vi "ctx get rssi value.vi"(9 "dest":u32, 10 "device_id":u32, 11 "context":u32) -> (1 "dest out":u32, 2 "function return":i32, 3 "context out":u32)   [LabVIEW 2019, in "apdm.lvlib"]
doc: "APDM_EXPORT int apdm_ctx_get_rssi_value(apdm_ctx_t context, const uint32_t device_id, uint32_t *dest);"
uses:
  apdm.lvlib
  Lee Lab/CP FES Walking 2018/Code/Working/LabVIEW/apdm.dll
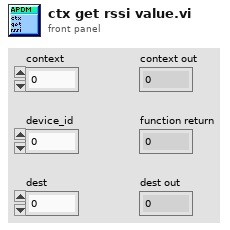
[diagram p1: front panel]
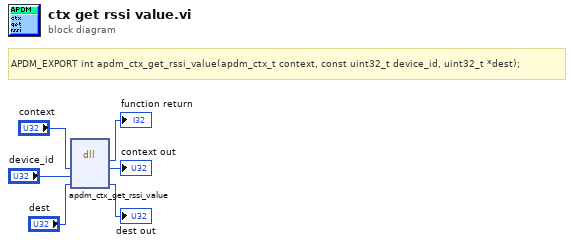
[diagram p0: block diagram]
diagram:
  # "APDM_EXPORT int apdm_ctx_get_rssi_value(apdm_ctx_t context, const uint32_t device_id, uint32_t *dest);"
  n1 = dll-call lib="C:/Users/jfalesi/Dropbox/Lee Lab/CP FES Walking 2018/Code/Working/LabVIEW/apdm.*" fn="apdm_ctx_get_rssi_value"("context"="context", "device_id"="device_id", "dest"="dest") -> (→"function return":i32, "context"=→"context out":u32, "dest"=→"dest out":u32)  [unwired: 4 in, 2 out]
